vi "FPGA IO.vi"() -> ()   [LabVIEW 2014]
uses:
  <vilib>/rvi/Emulation/niFpgaGetClockAttributes.vi
  <vilib>/rvi/Emulation/niFpgaSctlEmulationGetInTimedLoop.vi
  <vilib>/rvi/Emulation/niFpgaEmulationReportErrorSimple.vi
  <vilib>/rvi/eio/common/nirviEmuTemplateMethod_errors.vi
  <vilib>/rvi/Emulation/niFpgaCriticalErrorInLSC.vi
  <vilib>/eio/EIONode/EIONode.xnode
panel:
  in  "CW":bool
  in  "Move":bool
  in  "Width(uSec)":u32=500
  in  "Period(uSec))":u32=1000 caption="Period(uSec)"
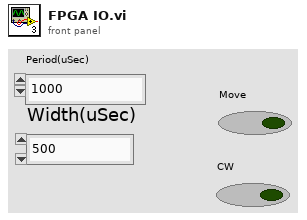
[diagram p1: front panel]
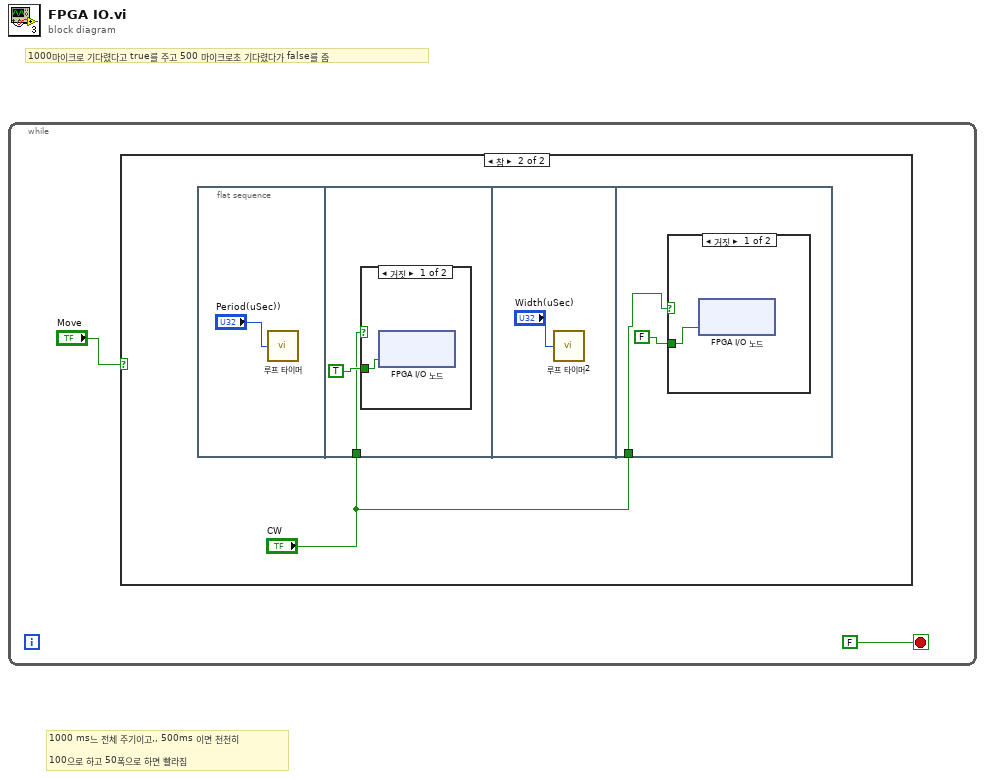
[diagram p0: block diagram]
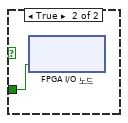
[diagram p3: hidden frame]
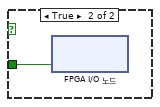
[diagram p4: hidden frame]
diagram:
  # "1000 ms느 전체 주기이고,, 500ms 이면 천천히\n\n100으로 하고 50폭으로 하면 빨라짐"
  # "1000마이크로 기다렸다고 true를 주고 500 마이크로초 기다렸다가 false를 줌"
  n1 = while {
    stop <- FALSE stop-if-true
    n2 = case shown="참" "Move" {
      frame False {
      }
      frame True {
        n3 = flat-sequence {
          tunnel: "CW" -> [w5]
          tunnel: "CW" -> [w10]
          frame #0 {
            n4 = call "루프 타이머"("Count(uSec)"="Period(uSec))") -> ()  [unwired: 1 out]
          }
          frame #1 {
            n5 = case shown="거짓" w5 {
              tunnel: TRUE ("CW") -> [w7 w8]
              frame False {
                n6 = xnode "FPGA I/O 노드"("CCW"=w7) -> ()  [unwired: 1 in, 1 out]
              }
              frame True {
                n7 = xnode "FPGA I/O 노드"("CW"=w8) -> ()  [unwired: 1 in, 1 out]
              }
            }
          }
          frame #2 {
            n8 = call "루프 타이머2"("Count(uSec)"="Width(uSec)") -> ()  [unwired: 1 out]
          }
          frame #3 {
            n9 = case shown="거짓" w10 {
              tunnel: FALSE ("CCW") -> [w12 w13]
              frame False {
                n10 = xnode "FPGA I/O 노드"("CCW"=w12) -> ()  [unwired: 1 in, 1 out]
              }
              frame True {
                n11 = xnode "FPGA I/O 노드"("CW"=w13) -> ()  [unwired: 1 in, 1 out]
              }
            }
          }
        }
      }
    }
  }
